vi "Driver VI Template Name.vi"(11 "CD Template":refnum<class "NIVS_CD Template.lvclass">) -> (2 "Driver VI Template Name":string)   [LabVIEW 2017, in "NIVS_CD Template.lvclass"]
uses:
  NIVS_CD Template.lvclass
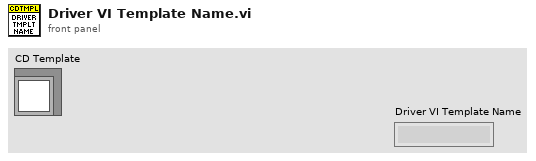
[diagram p1: front panel]
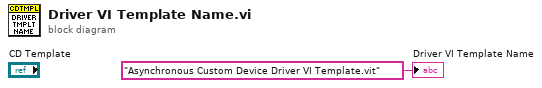
[diagram p0: block diagram]
diagram:
  "Driver VI Template Name" <- "Asynchronous Custom Device Driver VI Template.vit" ("Driver VI Template Name")
